vi "StringTStoTimeStamp.vi"() -> ()   [LabVIEW 2016, in "MiddlewareSALThisComponent.lvclass"]
uses:
  MiddlewareSALThisComponent.lvclass
panel:
  in  "TimeStamp":string
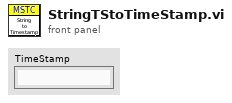
[diagram p1: front panel]
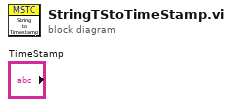
[diagram p0: block diagram]
diagram:
